vi "FGV Passwortlevel.vi"(6 "FGV Passwort Aktion":T2, 10 "Passworte neu":T1, 11 "geforderter Level":i16) -> (0 "Freigabe":bool, 2 "Passworte":T1, 3 "aktueller Level":i16)   [LabVIEW 2020, in "Passwort.lvlib"]
uses:
  Passwort.lvlib
  FGV Passwort Aktion.ctl
  Passwort Array.ctl
  Allgemein/allgemeine Sub-VIs.lvlib
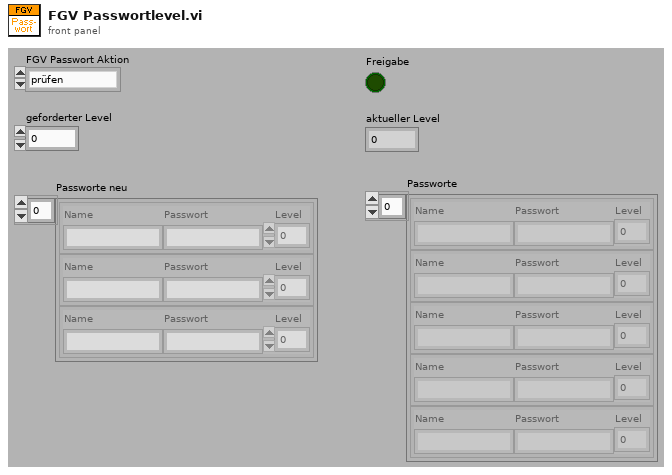
[diagram p1: front panel]
types:
  T1 = typedef "Passwort.lvlib/Passwort Array.ctl" = cluster{"Name":string, "Passwort":string, "Level":i16}[]
  T2 = typedef "Passwort.lvlib/FGV Passwort Aktion.ctl" = enum16{"prüfen", "setzen", "Initialisieren", "PW speichern", "lesen", "PW Änderung"}
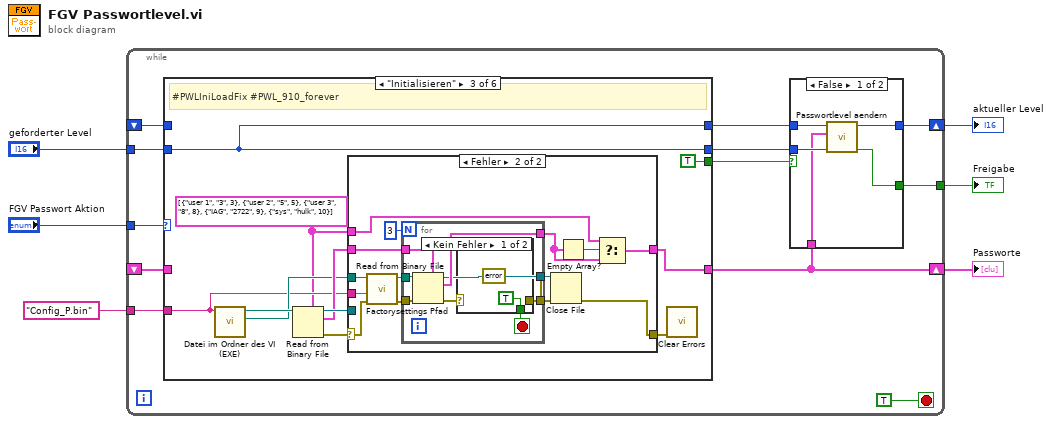
[diagram p0: block diagram]
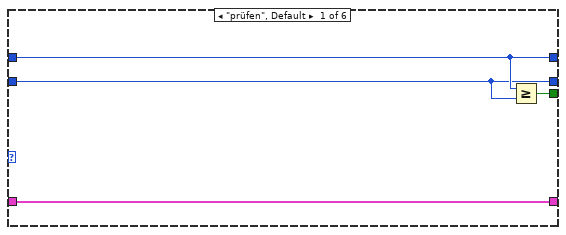
[diagram p3: hidden frame]
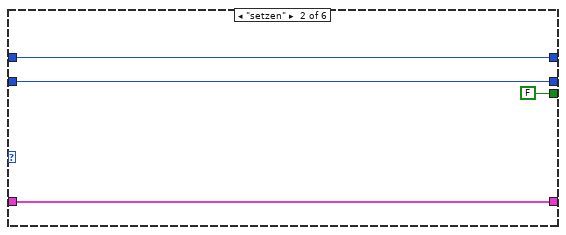
[diagram p4: hidden frame]
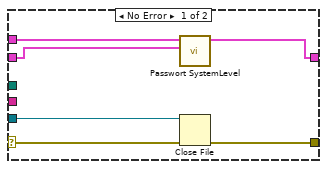
[diagram p5: hidden frame]
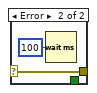
[diagram p6: hidden frame]
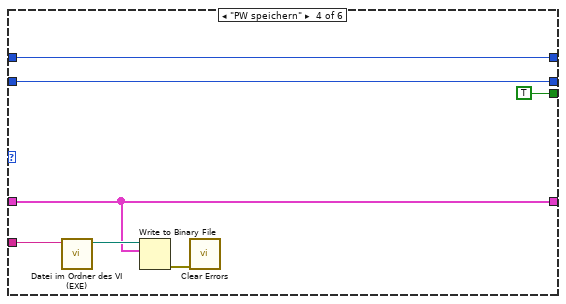
[diagram p7: hidden frame]
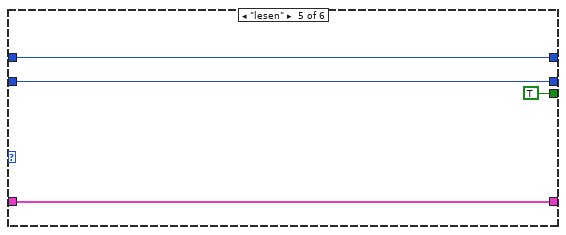
[diagram p8: hidden frame]
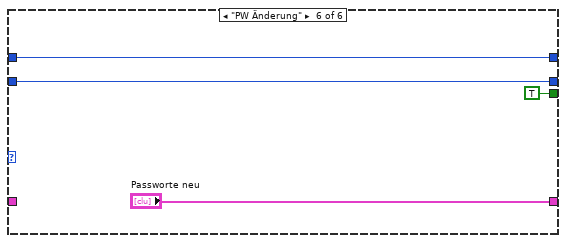
[diagram p9: hidden frame]
diagram:
  n1 = while {
    shift-right: [w11] -> w6
    shift-left: _ -> [w17]
    tunnel: "FGV Passwort Aktion" -> [w18]
    tunnel: "geforderter Level" -> [w15]
    tunnel: [w13] -> w4
    shift-right: [w8] -> w1
    shift-left: _ -> [w9]
    tunnel: "Config_P.bin" ("Dateiname") -> [w7]
    stop <- TRUE stop-if-true
    n2 = case shown="\"Initialisieren\"" w18 {
      tunnel: [w28 w32 w43 w83 w86 w90] -> w12
      tunnel: w17 -> [w28 w32 _ w83 w86 w90]
      tunnel: w15 -> [w27 w31 w43 w82 w85 w89]
      tunnel: [w29 FALSE TRUE TRUE TRUE TRUE] -> w14
      tunnel: [w27 w31 w43 w82 w85 w89] -> w10
      tunnel: [w26 w30 w36 w78 w84 "Passworte neu"] -> w8
      tunnel: w9 -> [w26 w30 _ w78 w84 _]
      tunnel: w7 -> [_ _ w37 w79 _ _]
      frame "prüfen", Default {
        n3 = Greater Or Equal?(x=w28, y=w27) -> (x >= y?=w29:bool)
      }
      frame "setzen" {
      }
      frame "Initialisieren" {
        w34 = T1 [{"Name"="user 1", "Passwort"="3", "Level"=3}, {"Name"="user 2", "Passwort"="5", "Level"=5}, {"Name"="user 3", "Passwort"="8", "Level"=8}, {"Name"="IAG", "Passwort"="2722", "Level"=9}, {"Name"="sys", "Passwort"="hulk", "Level"=10}] ("Passworte")
        # "#PWLIniLoadFix #PWL_910_forever"
        n4 = call "Datei im Ordner des VI (EXE).vi"("Dateiname"=w37) -> ("Ordner des Haupt-VIs"=w38:path, "Dateipfad im Ordner des Haupt-VIs"=w42:path)  [unwired: 8 in, 1 out]
        n5 = Read from Binary File(5:w34, 11:w42) -> (0:w41:errorcluster, 2:w39:T1, 3:w40:refnum<file>)  [unwired: 1 in, 4 out]
        n6 = case shown="Fehler" w41 {
          selector: w41 -> [w50 w57]
          tunnel: w38 -> [_ w58]
          tunnel: w39 -> [w46 w56]
          tunnel: [w47 w51] -> w36
          tunnel: [w48 w62] -> w35
          tunnel: w40 -> [w49 _]
          tunnel: w37 -> [_ w55]
          tunnel: w34 -> [w45 w53]
          frame No Error {
            n7 = call "Passwort SystemLevel.vi"("Passworte gelesen"=w46, "Default Passworte"=w45) -> ("Passworte"=w47:T1)  [unwired: 9 in]
            n8 = Close File(refnum=w49, error in=w50) -> (error out=w48:errorcluster)  [unwired: 1 out]
          }
          frame Error {
            n9 = call "Factorysettings Pfad.vi"("error in (no error)"=w57, "Dateiname"=w55, "Ordner des Haupt-VIs"=w58) -> ("error out"=w59:errorcluster, "Pfad Factorysettings"=w60:path)  [unwired: 7 in]
            n10 = for {
              N: 3 -> [_]
              tunnel: w59 -> [w70]
              tunnel: w60 -> [w69]
              tunnel: [w68] -> w52
              tunnel: [w67] -> w63
              tunnel: [w66] -> w61
              tunnel: w56 -> [w65]
              stop <- w71 stop-if-true
              n11 = Read from Binary File(5:w65, 8:w70, 11:w69) -> (0:w72:errorcluster, 2:w68:T1, 3:w66:refnum<file>)  [unwired: 3 in, 1 out]
              n12 = case shown="Kein Fehler" w72 {
                selector: w72 -> [_ w75]
                tunnel: [TRUE _] -> w71
                tunnel: [errorcluster {"status"=FALSE, "code"=0, "source"=""} ("error IO") w75] -> w67
                frame No Error {
                }
                frame Error {
                  n13 = Wait (ms)(milliseconds to wait=u32 100 ("Zu wartende ms")) -> ()  [unwired: 1 out]
                }
              }
            }
            n14 = Close File(refnum=w61, error in=w63) -> (error out=w62:errorcluster)  [unwired: 1 out]
            n15 = Empty Array?(array=w52) -> (empty?=w54:bool)
            n16 = Select(t=w53, s=w54, f=w52) -> (s? t:f=w51:T1)
          }
        }
        n17 = call <vilib>:"Clear Errors.vi"("error in (no error)"=w35) -> ()  [unwired: 5 in, 2 out]
      }
      frame "PW speichern" {
        n18 = call "Datei im Ordner des VI (EXE).vi"("Dateiname"=w79) -> ("Dateipfad im Ordner des Haupt-VIs"=w80:path)  [unwired: 8 in, 2 out]
        n19 = Write to Binary File(file (use dialog)=w80, data=w78) -> (error out=w77:errorcluster)  [unwired: 1 in, 5 out]
        n20 = call <vilib>:"Clear Errors.vi"("error in (no error)"=w77) -> ()  [unwired: 5 in, 2 out]
      }
      frame "lesen" {
      }
      frame "PW Änderung" {
      }
    }
    n21 = case shown="False" w14 {
      selector: w14 -> [_ w25]
      tunnel: [w23 w25] -> w13
      tunnel: w12 -> [w20 w24]
      tunnel: [w21 w24] -> w11
      tunnel: w10 -> [w22 _]
      tunnel: w8 -> [w19 _]
      frame False {
        n22 = call "Passwortlevel aendern.vi"("geforderter Level"=w22, "Passworte"=w19, "aktueller Level"=w20) -> ("Freigabe"=w23:bool, "aktueller Level"=w21:i16)  [unwired: 7 out]
      }
      frame True {
        # "Freigabe"
      }
    }
  }
  "aktueller Level" <- w6
  "Freigabe" <- w4
  "Passworte" <- w1
